vi "icListen 2 Position.vi"() -> ()   [LabVIEW 2020, in "PAM Library.lvlib"]
uses:
  PAM Library.lvlib
panel:
  in  "icListen 2 Position":string
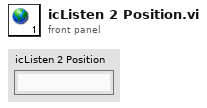
[diagram p1: front panel]
diagram:
